vi "CPU_SP_pop.vi"(11 "registers":T1 {"P" format="%08b"; "PC" format="%04x"; "SP" format="%02x"; "Y" format="%02x"; "X" format="%02x"; "A" format="%02x"}) -> (2 "value":u8 format="%02x", 3 "registers":T1 {"P" format="%08b"; "PC" format="%04x"; "SP" format="%02x"; "Y" format="%02x"; "X" format="%02x"; "A" format="%02x"})   [LabVIEW 2018]
uses:
  CPU_registers.ctl
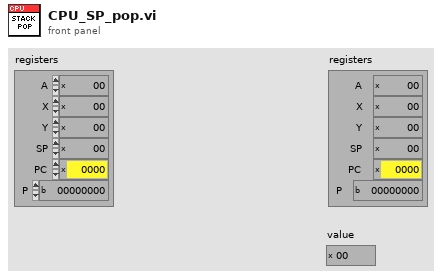
[diagram p1: front panel]
types:
  T1 = typedef "CPU_registers.ctl" = cluster{"A":u8, "X":u8, "Y":u8, "SP":u8, "PC":u16, "P":u8}
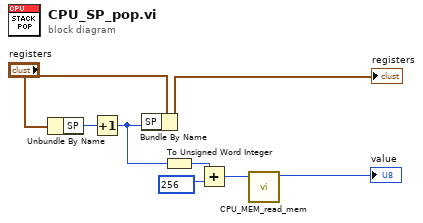
[diagram p0: block diagram]
diagram:
  n1 = Unbundle By Name("registers") -> ("SP"=w6:u8)
  n2 = Increment(x=w6) -> (x+1=w2:u8)
  n3 = Bundle By Name(cluster="registers", "SP"=w2) -> (→"registers":T1)
  n4 = To Unsigned Word Integer(number=w2) -> (unsigned 16bit integer=w7:u16)
  n5 = Add(x=w7, y=u16 256) -> (x+y=w3:u16)
  n6 = call "CPU_MEM_read_mem.vi"("address"=w3) -> ("value out"=→"value":u8)  [unwired: 10 in]
